vi "setPower.vi"(8 "error in (no error)":errorcluster, 9 "Channel":i32, 10 "Power (dBm)":dbl, 11 "Instrument.VSource in":refnum<class "Instrument.VNA.lvclass">) -> (0 "error out":errorcluster, 3 "Instrument.VSource out":refnum<class "Instrument.VNA.lvclass">)   [LabVIEW 2019, in "Instrument.VNA.lvclass"]
uses:
  Instrument.VNA.lvclass
  Typedefs/setPower--cluster.ctl
  Typedefs/VNA.Commands--Enum.ctl
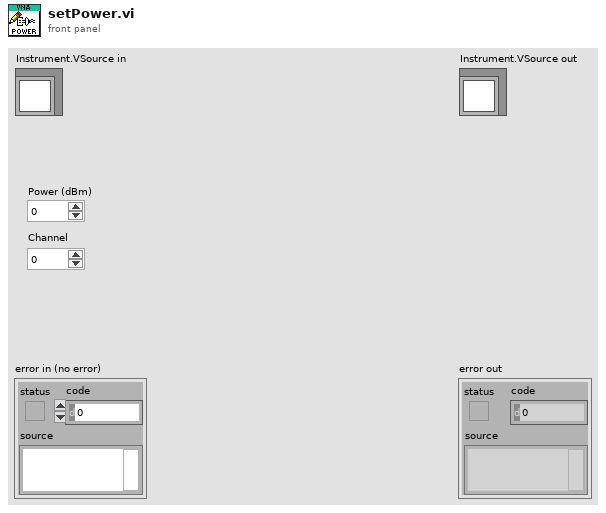
[diagram p1: front panel]
types:
  T1 = typedef "Instrument.VNA.lvclass/VNA.Commands--Enum.ctl" = enum16{"getData", "setAverage", "setFormat", "setMeasurement", "setPower", "setSweep"}
  T2 = typedef "Instrument.VNA.lvclass/setPower--cluster.ctl" = cluster{"power":dbl, "channel":i32}
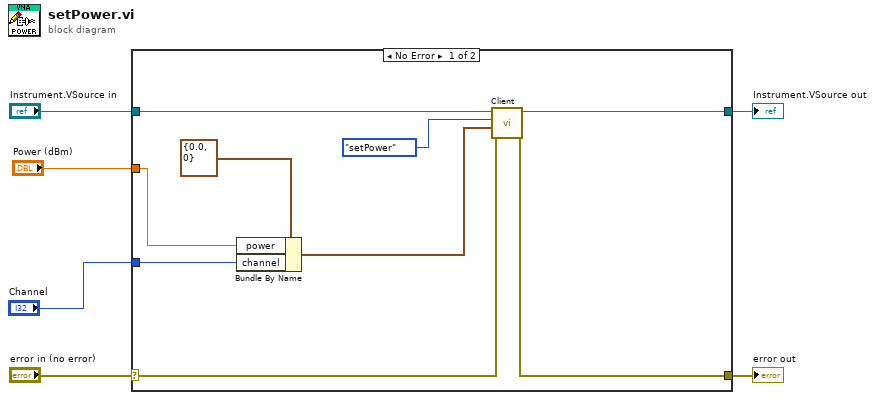
[diagram p0: block diagram]
diagram:
  n1 = case shown="No Error" "error in (no error)" {
    selector: "error in (no error)" -> [w8 w17]
    tunnel: [w10 w17] -> w5
    tunnel: [w14 w16] -> w3
    tunnel: "Instrument.VSource in" -> [w9 w16]
    tunnel: "Power (dBm)" -> [w12 _]
    tunnel: "Channel" -> [w11 _]
    frame No Error {
      n2 = Bundle By Name(cluster=T2 {"power"=0.0, "channel"=0} ("setPower"), "power"=w12, "channel"=w11) -> (w15:T2)
      n3 = call-dynamic "Client.vi"("error in (no error)"=w8, "Data in"=w15, "Command in"=VNA.Commands--Enum."setPower" ("Commands"), "Instrument in"=w9) -> ("error out"=w10:errorcluster, "Instrument out"=w14:refnum<class "Instrument.VNA.lvclass">)  [unwired: 4 in, 2 out]
    }
    frame Error {
    }
  }
  "error out" <- w5
  "Instrument.VSource out" <- w3
